vi "readTcpPackets.vi"(8 "error in (no error)":errorcluster, 10 "timeout ms":i32=1000, 11 "connection ID in":refnum<k5>) -> (0 "error out":errorcluster, 2 "TCP packets":string[](array[string]), 3 "connection ID out":refnum<k5>, 4 "seconds":dbl, 6 "rate (Hz)":dbl format="%#_4f")   [LabVIEW 2018]
doc: "Read TCP packets comming from TCP server."
panel:
  out "size(s)":i32
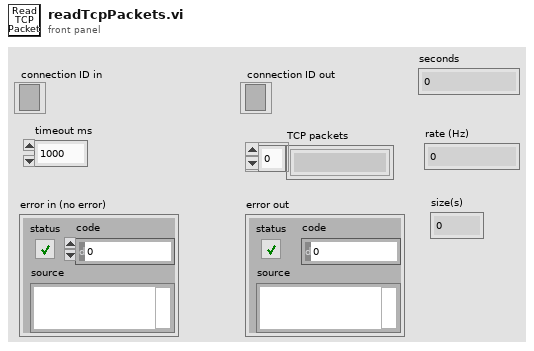
[diagram p1: front panel]
types:
  T1 = enum16{"Standard", "Buffered", "CRLF", "Immediate"}
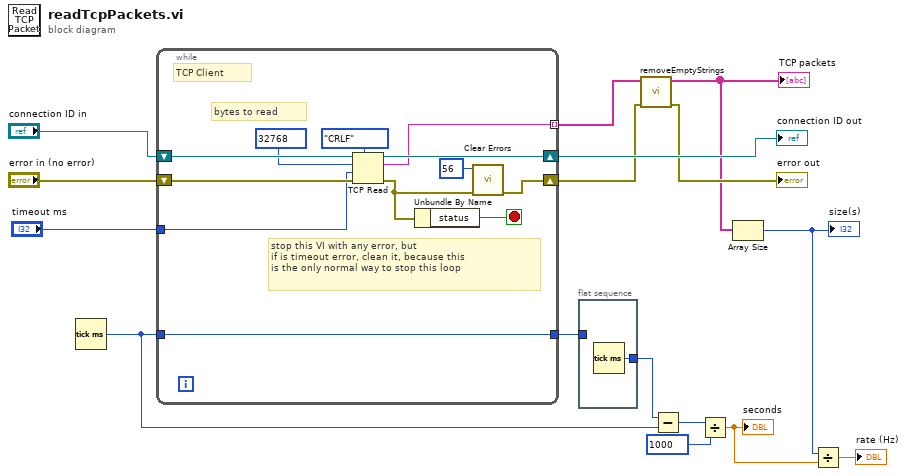
[diagram p0: block diagram]
diagram:
  n1 = Tick Count (ms)() -> (millisecond timer value=w9:u32)
  n2 = while {
    shift-right: [w26] -> w16
    shift-left: "connection ID in" -> [w28]
    shift-right: [w23] -> w13
    shift-left: "error in (no error)" -> [w27]
    tunnel: [w21] -> w3 mode=indexing
    tunnel: "timeout ms" -> [w18]
    tunnel: w9 -> [w17]
    tunnel: [w17] -> w8
    stop <- w19 stop-if-true
    # "bytes to read"
    # "stop this VI with any error, but\nif is timeout error, clean it, because this\nis the only normal way to stop this loop"
    # "TCP Client"
    n3 = TCP Read(connection ID=w28, bytes to read=32768, error in (no error)=w27, 7:T1."CRLF" ("mode (standard)"), 9:w18) -> (connection ID out=w26:refnum<k5>, data out=w21:string, error out=w20:errorcluster)
    n4 = Unbundle By Name(w20) -> ("status"=w19:bool)
    n5 = call <vilib>:"Clear Errors.vi"("error in (no error)"=w20, "specific error code to clear (0: all)"=56) -> ("error out"=w23:errorcluster)  [unwired: 4 in, 1 out]
  }
  "connection ID out" <- w16
  n6 = flat-sequence {
    tunnel: [w29] -> w10
    tunnel: w8 -> [_]
    frame #0 {
      n7 = Tick Count (ms)() -> (millisecond timer value=w29:u32)
    }
  }
  n8 = call "removeEmptyStrings.vi"("error in (no error)"=w13, "stringArray in"=w3) -> ("error out"=→"error out":errorcluster, "stringArray out"=w2:string[])  [unwired: 8 in]
  "TCP packets" <- w2
  n9 = Subtract(x=w10, y=w9) -> (x-y=w7:u32)
  n10 = Divide(x=w7, y=u32 1000) -> (x/y=w5:dbl)
  "seconds" <- w5
  n11 = Array Size(array=w2) -> (size(s)=w1:i32)
  "size(s)" <- w1
  n12 = Divide(x=w1, y=w5) -> (x/y=→"rate (Hz)":dbl)
